vi "DisplayImage.vi"(0 "frame":T1, 1 "ImageIMAQ":T2, 2 "PixelPointerIn":u64, 5 "Image Display Refnum":refnum<vi>) -> (6 "frame":T1, 7 "PixelPointerOut":u64)   [LabVIEW 2019]
uses:
  <vilib>/vision/Image Controls.llb/IMAQ Image.ctl
  <resource>/objmgr/IMAQImage.rc
  EmergentCameraC/EmergentCameraC.lvlib
panel:
  out "WidthImageIMAQStatic":u32
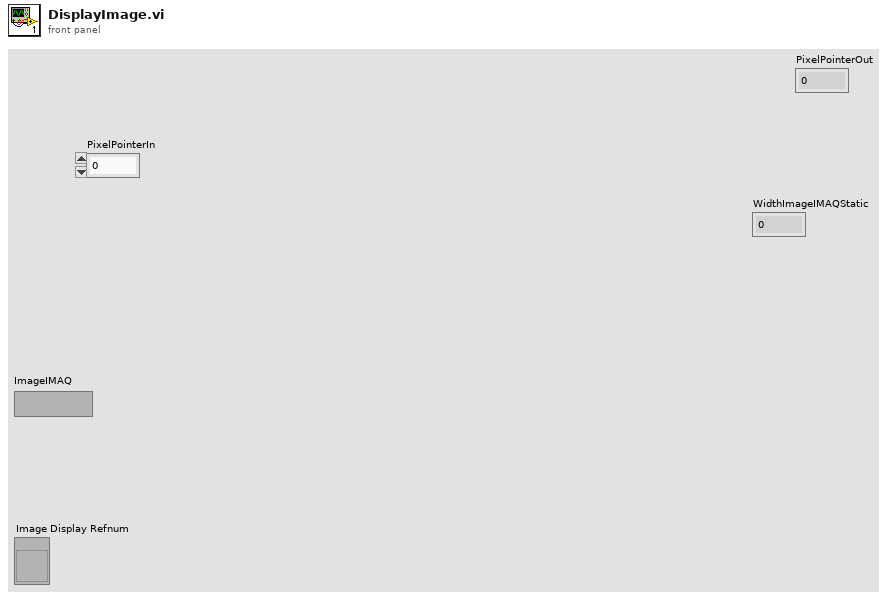
[diagram p1: front panel]
types:
  T1 = cluster{"pixel_type":u32, "size_x":u32, "size_y":u32, "stride":i32, "offset_x":u32, "offset_y":u32, "padding_x":u32, "padding_y":u32, "trailer_size_y":u32, "frame_id":u16, "@dummy control@":i8, "@dummy control@":i8, "imagePtr":i64, "bufferSize":u32, "@dummy control@":i8, "@dummy control@":i8, "@dummy control@":i8, "@dummy control@":i8, "timestamp":u64, "nsecs":u64, "convertColor":i32, "convertBitDepth":i32, "privateData[0]":u8, "privateData[1]":u8, "privateData[2]":u8, "privateData[3]":u8, "privateData[4]":u8, "privateData[5]":u8, "privateData[6]":u8, "privateData[7]":u8, "privateData[8]":u8, "privateData[9]":u8, "privateData[10]":u8, "privateData[11]":u8, "privateData[12]":u8, "privateData[13]":u8, "privateData[14]":u8, "privateData[15]":u8, "privateData[16]":u8, "privateData[17]":u8, "privateData[18]":u8, "privateData[19]":u8, "privateData[20]":u8, "privateData[21]":u8, "privateData[22]":u8, "privateData[23]":u8, "privateData[24]":u8, "privateData[25]":u8, "privateData[26]":u8, "privateData[27]":u8, "privateData[28]":u8, "privateData[29]":u8, "privateData[30]":u8, "privateData[31]":u8, "privateData[32]":u8, "privateData[33]":u8, "privateData[34]":u8, "privateData[35]":u8, "privateData[36]":u8, "privateData[37]":u8, "privateData[38]":u8, "privateData[39]":u8, "privateData[40]":u8, "privateData[41]":u8, "privateData[42]":u8, "privateData[43]":u8, "privateData[44]":u8, "privateData[45]":u8, "privateData[46]":u8, "privateData[47]":u8, "privateData[48]":u8, "privateData[49]":u8, "privateData[50]":u8, "privateData[51]":u8, "privateData[52]":u8, "privateData[53]":u8, "privateData[54]":u8, "privateData[55]":u8, "privateData[56]":u8, "privateData[57]":u8, "privateData[58]":u8, "privateData[59]":u8, "privateData[60]":u8, "privateData[61]":u8, "privateData[62]":u8, "privateData[63]":u8, "privateData[64]":u8, "privateData[65]":u8, "privateData[66]":u8, "privateData[67]":u8, "privateData[68]":u8, "privateData[69]":u8, "privateData[70]":u8, "privateData[71]":u8, "privateData[72]":u8, "privateData[73]":u8, "privateData[74]":u8, "privateData[75]":u8, "privateData[76]":u8, "privateData[77]":u8, "privateData[78]":u8, "privateData[79]":u8, "privateData[80]":u8, "privateData[81]":u8, "privateData[82]":u8, "privateData[83]":u8, "privateData[84]":u8, "privateData[85]":u8, "privateData[86]":u8, "privateData[87]":u8, "privateData[88]":u8, "privateData[89]":u8, "privateData[90]":u8, "privateData[91]":u8, "privateData[92]":u8, "privateData[93]":u8, "privateData[94]":u8, "privateData[95]":u8, "privateData[96]":u8, "privateData[97]":u8, "privateData[98]":u8, "privateData[99]":u8, "privateData[100]":u8, "privateData[101]":u8, "privateData[102]":u8, "privateData[103]":u8, "privateData[104]":u8, "privateData[105]":u8, "privateData[106]":u8, "privateData[107]":u8, "privateData[108]":u8, "privateData[109]":u8, "privateData[110]":u8, "privateData[111]":u8, "privateData[112]":u8, "privateData[113]":u8, "privateData[114]":u8, "privateData[115]":u8, "privateData[116]":u8, "privateData[117]":u8, "privateData[118]":u8, "privateData[119]":u8, "privateData[120]":u8, "privateData[121]":u8, "privateData[122]":u8, "privateData[123]":u8, "privateData[124]":u8, "privateData[125]":u8, "privateData[126]":u8, "privateData[127]":u8, "privateData[128]":u8, "privateData[129]":u8, "privateData[130]":u8, "privateData[131]":u8, "privateData[132]":u8, "privateData[133]":u8, "privateData[134]":u8, "privateData[135]":u8, "privateData[136]":u8, "privateData[137]":u8, "privateData[138]":u8, "privateData[139]":u8, "privateData[140]":u8, "privateData[141]":u8, "privateData[142]":u8, "privateData[143]":u8, "privateData[144]":u8, "privateData[145]":u8, "privateData[146]":u8, "privateData[147]":u8, "privateData[148]":u8, "privateData[149]":u8, "privateData[150]":u8, "privateData[151]":u8, "privateData[152]":u8, "privateData[153]":u8, "privateData[154]":u8, "privateData[155]":u8, "privateData[156]":u8, "privateData[157]":u8, "privateData[158]":u8, "privateData[159]":u8, "privateData[160]":u8, "privateData[161]":u8, "privateData[162]":u8, "privateData[163]":u8, "privateData[164]":u8, "privateData[165]":u8, "privateData[166]":u8, "privateData[167]":u8, "privateData[168]":u8, "privateData[169]":u8, "privateData[170]":u8, "privateData[171]":u8, "privateData[172]":u8, "privateData[173]":u8, "privateData[174]":u8, "privateData[175]":u8, "privateData[176]":u8, "privateData[177]":u8, "privateData[178]":u8, "privateData[179]":u8, "privateData[180]":u8, "privateData[181]":u8, "privateData[182]":u8, "privateData[183]":u8, "privateData[184]":u8, "privateData[185]":u8, "privateData[186]":u8, "privateData[187]":u8, "privateData[188]":u8, "privateData[189]":u8, "privateData[190]":u8, "privateData[191]":u8, "privateData[192]":u8, "privateData[193]":u8, "privateData[194]":u8, "privateData[195]":u8, "privateData[196]":u8, "privateData[197]":u8, "privateData[198]":u8, "privateData[199]":u8, "privateData[200]":u8, "privateData[201]":u8, "privateData[202]":u8, "privateData[203]":u8, "privateData[204]":u8, "privateData[205]":u8, "privateData[206]":u8, "privateData[207]":u8, "privateData[208]":u8, "privateData[209]":u8, "privateData[210]":u8, "privateData[211]":u8, "privateData[212]":u8, "privateData[213]":u8, "privateData[214]":u8, "privateData[215]":u8, "privateData[216]":u8, "privateData[217]":u8, "privateData[218]":u8, "privateData[219]":u8, "privateData[220]":u8, "privateData[221]":u8, "privateData[222]":u8, "privateData[223]":u8, "privateData[224]":u8, "privateData[225]":u8, "privateData[226]":u8, "privateData[227]":u8, "privateData[228]":u8, "privateData[229]":u8, "privateData[230]":u8, "privateData[231]":u8, "privateData[232]":u8, "privateData[233]":u8, "privateData[234]":u8, "privateData[235]":u8, "privateData[236]":u8, "privateData[237]":u8, "privateData[238]":u8, "privateData[239]":u8, "privateData[240]":u8, "privateData[241]":u8, "privateData[242]":u8, "privateData[243]":u8, "privateData[244]":u8, "privateData[245]":u8, "privateData[246]":u8, "privateData[247]":u8, "privateData[248]":u8, "privateData[249]":u8, "privateData[250]":u8, "privateData[251]":u8, "privateData[252]":u8, "privateData[253]":u8, "privateData[254]":u8, "privateData[255]":u8}
  T2 = typedef "IMAQ Image.ctl" = refnum<image>
  T3 = enum32{"Map Pixel Pointer", "Unmap Pixel Pointer", "Get Pixels Infos"}
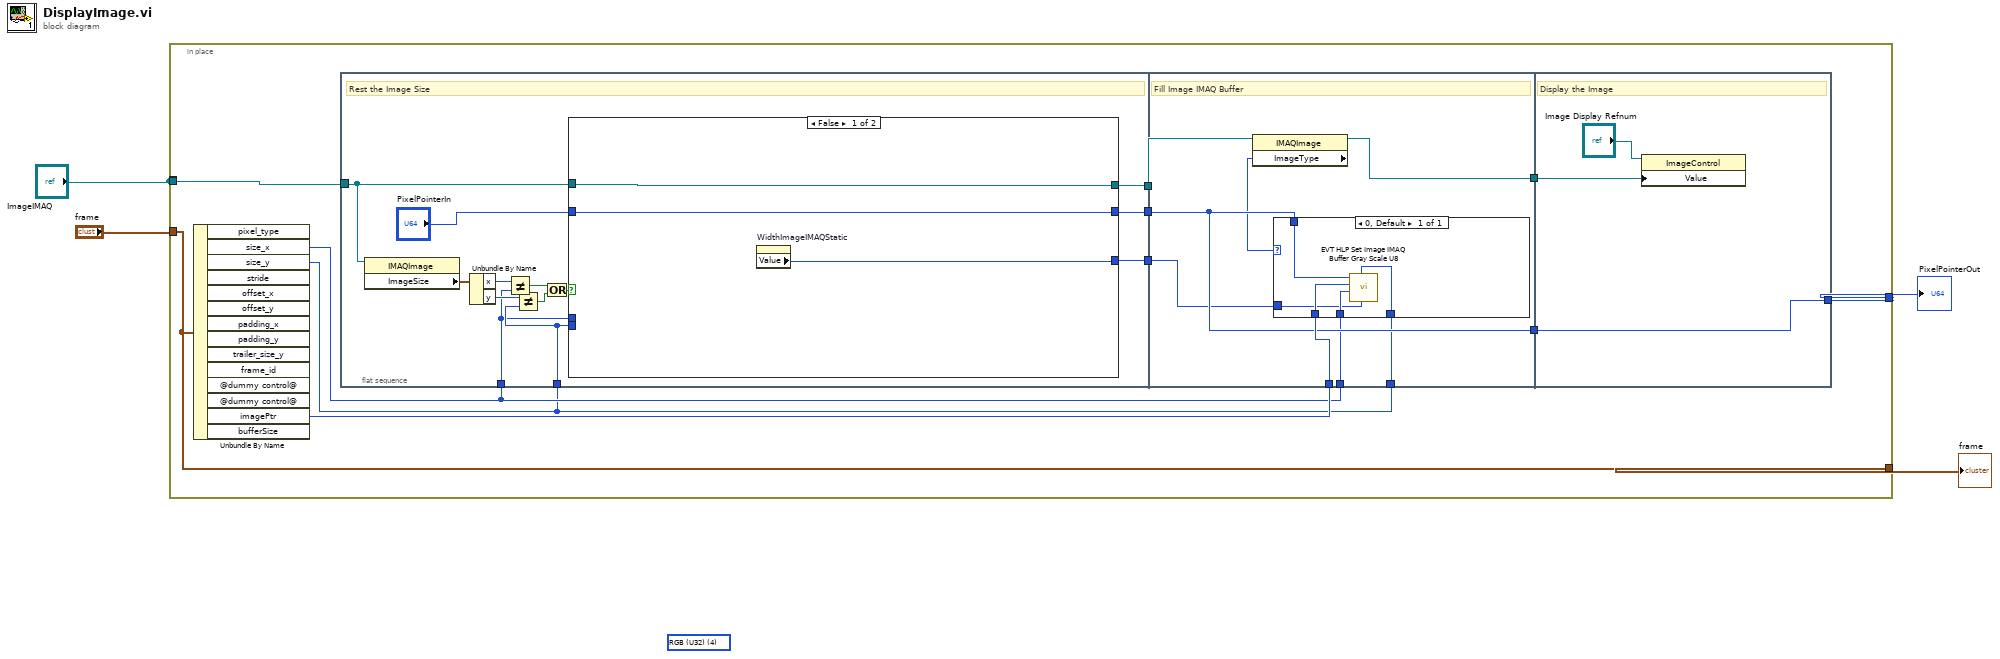
[diagram p0: block diagram]
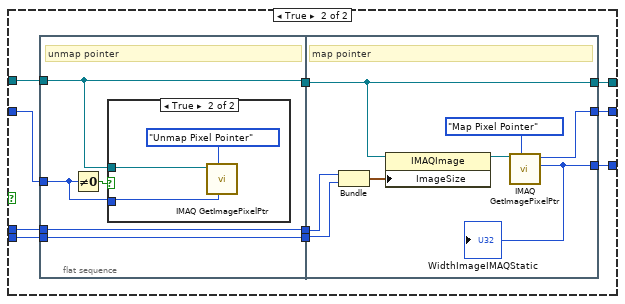
[diagram p2: hidden frame]
diagram:
  (unwired) u32 4 items=["Grayscale (U8)", "Grayscale (I16)", "Grayscale (SGL)", "Complex (CSG)", "RGB (U32)", "HSL (U32)", "RGB (U64)", "Grayscale (U16)"] ("Image Type")
  n1 = in-place {
    in-place-border: "frame" -> [w15]
    in-place-border: [w15] -> w3
    in-place-border: "ImageIMAQ" -> [_]
    in-place-border: "ImageIMAQ" -> [w12]
    in-place-border: [w9] -> w1
    n2 = Unbundle By Name(w15) -> ("size_x"=w6:u32, "size_y"=w5:u32, "imagePtr"=w10:i64)  [unwired: 11 out]
    n3 = flat-sequence {
      tunnel: [w20] -> w14
      tunnel: w6 -> [w21]
      tunnel: w5 -> [w22]
      tunnel: [w19] -> w13
      tunnel: w12 -> [w18]
      tunnel: [w16] -> w7
      tunnel: w14 -> [w62]
      tunnel: w13 -> [w64]
      tunnel: [w63] -> w11
      tunnel: w10 -> [w65]
      tunnel: [w64] -> w8
      tunnel: w7 -> [w60]
      tunnel: w6 -> [w59]
      tunnel: w5 -> [w58]
      tunnel: w11 -> [w73]
      tunnel: [w71] -> w9
      tunnel: w8 -> [w71]
      frame #0 {
        # "Rest the Image Size"
        n4 = property class="IMAQImage"(reference=w18) -> ("ImageSize"=w28:cluster{"x":i32, "y":i32})  [unwired: 1 in, 2 out]
        n5 = Unbundle By Name(w28) -> ("x"=w27:i32, "y"=w26:i32)
        n6 = Not Equal?(x=w27, y=w21) -> (x != y?=w24:bool)
        n7 = Not Equal?(x=w26, y=w22) -> (x != y?=w25:bool)
        n8 = Or(x=w24, y=w25) -> (x .or. y?=w23:bool)
        n9 = case shown="False" w23 {
          tunnel: w22 -> [_ w36]
          tunnel: w21 -> [_ w38]
          tunnel: [w31 w35] -> w20
          tunnel: [w30 w34] -> w19
          tunnel: w18 -> [w31 w41]
          tunnel: "PixelPointerIn" -> [w30 w33]
          tunnel: [w29 w32] -> w16
          frame False {
            n10 = property on="WidthImageIMAQStatic" class="DigNum (strict)"() -> ("Value"=w29:u32)  [unwired: 2 in, 2 out]
          }
          frame True {
            n11 = flat-sequence {
              tunnel: w41 -> [w45]
              tunnel: [w45] -> w40
              tunnel: [w44] -> w39
              tunnel: w38 -> [w44]
              tunnel: [w43] -> w37
              tunnel: w36 -> [w43]
              tunnel: w33 -> [w42]
              tunnel: w40 -> [w52]
              tunnel: w39 -> [w54]
              tunnel: w37 -> [w53]
              tunnel: [w52] -> w35
              tunnel: [w51] -> w34
              tunnel: [w50] -> w32
              frame #0 {
                # "unmap pointer"
                n12 = Not Equal To 0?(x=w42) -> (x != 0?=w46:bool)
                n13 = case shown="True" w46 {
                  tunnel: w42 -> [_ w48]
                  tunnel: w45 -> [_ w47]
                  frame False {
                  }
                  frame True {
                    n14 = call "IMAQ GetImagePixelPtr"("Pixel Pointer in"=w48, "Function"=T3."Unmap Pixel Pointer", "Image"=w47) -> ()  [unwired: 3 in, 6 out]
                  }
                }
              }
              frame #1 {
                # "map pointer"
                n15 = Bundle("size_x"=w54, "size_y"=w53) -> (w55:cluster{"size_x":u32, "size_y":u32})  [unwired: 1 in]
                n16 = property class="IMAQImage"(reference=w52, "ImageSize"=w55) -> (reference out=w57:T2)  [unwired: 1 in, 1 out]
                n17 = call "IMAQ GetImagePixelPtr"("Function"=T3."Map Pixel Pointer", "Image"=w57) -> ("LineWidth(Pixels)"=w50:i32, "Pixel Pointer out"=w51:u64)  [unwired: 4 in, 4 out]
                "WidthImageIMAQStatic" <- w50
              }
            }
          }
        }
      }
      frame #1 {
        # "Fill Image IMAQ Buffer"
        n18 = property class="IMAQImage"(reference=w62) -> (reference out=w63:T2, "ImageType"=w61:u32)  [unwired: 1 in, 1 out]
        n19 = case shown="0, Default" w61 {
          tunnel: w65 -> [w70]
          tunnel: w64 -> [w69]
          tunnel: w60 -> [w66]
          tunnel: w59 -> [w68]
          tunnel: w58 -> [w67]
          frame 0, Default {
            n20 = call "EVT HLP Set Image IMAQ Buffer Gray Scale U8.vi"("widthLV"=w66, "height"=w67, "width"=w68, "srcBuffer"=w70, "IMAQbuffer"=w69) -> ()  [unwired: 7 in]
          }
        }
      }
      frame #2 {
        # "Display the Image"
        n21 = property class="ImageControl"(reference="Image Display Refnum", "Value"=w73) -> ()  [unwired: 1 in, 2 out]
      }
    }
  }
  "frame" <- w3
  "PixelPointerOut" <- w1
